vi "Save.vi"(0 "Grid in":refnum<class "Grid.lvclass">) -> (2 "error out":errorcluster, 3 "FileName":string, 4 "Grid out":refnum<class "Grid.lvclass">)   [LabVIEW 2016, in "Grid.lvclass"]
doc: "Save the IDs and Type of Neurons of all the active nodes (Neurons) inside the saving folder (\\Results Default) with the name of the class. Ask for overwriting."
uses:
  Grid.lvclass
  Grid.lvclass/Grid.ctl
  <vilib>/Utility/xml.llb/Write to XML File(string).vi
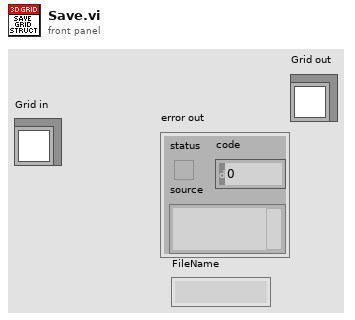
[diagram p1: front panel]
types:
  T1 = enum16{"open", "replace", "create", "open or create", "replace or create", "replace or create with confirmation"}
  T2 = typedef "Neuron Info.ctl" = cluster{"N":i32, "Radius":dbl, "Type":T3, "Color":u32}[]
  T3 = typedef "Type of Neuron.ctl" = enum16{"MF", "BA", "GO", "GC", "PC", "LU", "Glia (Dummy)"}
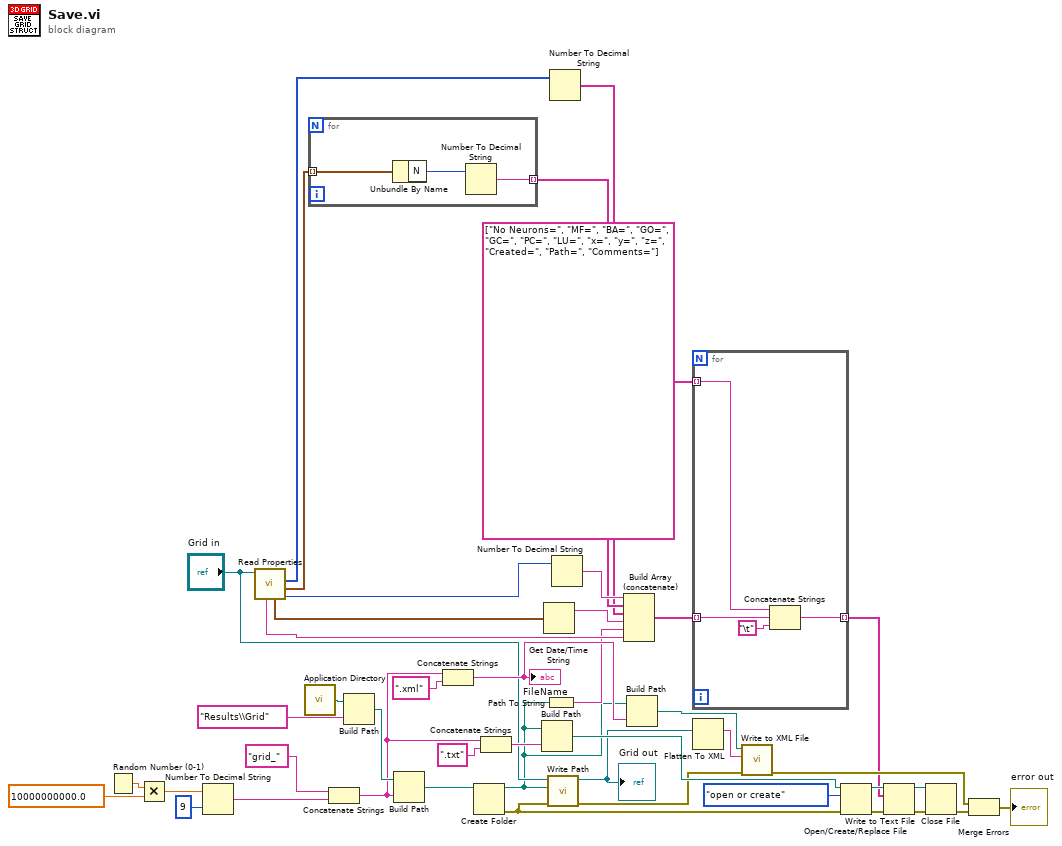
[diagram p0: block diagram]
diagram:
  n1 = Random Number (0-1)() -> (number: 0 to 1=w20:dbl)
  n2 = Multiply(x=w20, y=10000000000.0) -> (x*y=w18:dbl)
  n3 = Number To Decimal String(number=w18, width (-)=i16 9) -> (decimal integer string=w15:string)
  n4 = call "Read Properties.vi"("Grid in"="Grid in") -> ("No Neurons"=w37:i32, "Neurons Info"=w36:T2, "Size(um)"=w38:u32[], "Created at"=w22:timestamp, "Comments"=w7:string)  [unwired: 3 in, 3 out]
  n5 = call <vilib>:"Application Directory.vi"() -> ("Application Directory"=w44:path)
  n6 = for {
    tunnel: w36 -> [w47] mode=indexing
    tunnel: [w45] -> w34 mode=indexing
    n7 = Unbundle By Name(w47) -> ("N"=w46:i32)
    n8 = Number To Decimal String(number=w46) -> (decimal integer string=w45:string)  [unwired: 1 in]
  }
  n9 = Concatenate Strings("grid_" ("time format string (%c)"), w15) -> (w9:string)
  n10 = Build Path(base path=w44, name or relative path="Results\\Grid") -> (appended path=w14:path)
  n11 = Build Path(base path=w14, name or relative path=w9) -> (appended path=w8:path)
  n12 = Concatenate Strings(w9, ".xml" ("string")) -> (w13:string)
  "FileName" <- w13
  n13 = Create Folder(path (use dialog)=w8) -> (created path=w1:path, error out=w2:errorcluster)  [unwired: 2 in, 1 out]
  n14 = Concatenate Strings(w9, ".txt" ("string")) -> (w10:string)
  n15 = Build Path(base path=w1, name or relative path=w10) -> (appended path=w32:path)
  n16 = Get Date/Time String(seconds (now)=w22) -> (date string=w21:string)  [unwired: 2 in, 1 out]
  n17 = Path To String(path=w1) -> (string=w6:string)
  n18 = call-dynamic "Write Path.vi"("error in (no error)"=w2, "Path"=w1, "Grid in"="Grid in") -> ("error out"=w3:errorcluster, "Grid out"=w4:refnum<class "Grid.lvclass">)  [unwired: 7 in]
  "Grid out" <- w4
  n19 = Number To Decimal String(number=w38) -> (decimal integer string=w33:string[])  [unwired: 1 in]
  n20 = Number To Decimal String(number=w37) -> (decimal integer string=w35:string)  [unwired: 1 in]
  n21 = Build Array (concatenate)(w35, w34, w33, w21, w6, w7) -> (w25:string[])
  n22 = Build Path(base path=w1, name or relative path=w13) -> (appended path=w41:path)
  n23 = for {
    tunnel: w25 -> [w49] mode=indexing
    tunnel: [w51] -> w23 mode=indexing
    tunnel: string[] ["No Neurons=", "MF=", "BA=", "GO=", "GC=", "PC=", "LU=", "x=", "y=", "z=", "Created=", "Path=", "Comments="] -> [w50] mode=indexing
    n24 = Concatenate Strings(w50, w49, "\t") -> (w51:string)
  }
  n25 = Flatten To XML(anything=w4) -> (xml string=w42:string)
  n26 = call-poly <vilib>:"Write to XML File.vi"("error in (no error)"=w3, "XML Input"=w42, "XML File Path"=w41) -> ("error out"=w39:errorcluster)  [unwired: 6 in, 2 out]
  n27 = Open/Create/Replace File(file path (use dialog)=w32, error in=w2, operation (0:open)=T1."open or create") -> (refnum out=w30:refnum<file>, error out=w31:errorcluster)  [unwired: 3 in, 1 out]
  n28 = Write to Text File(file (use dialog)=w30, text=w23, error in=w31) -> (refnum out=w29:refnum<file>, error out=w28:errorcluster)  [unwired: 1 in, 1 out]
  n29 = Close File(refnum=w29, error in=w28) -> (error out=w27:errorcluster)  [unwired: 1 out]
  n30 = Merge Errors(w39, w27) -> (→"error out":errorcluster)
